vi "loop_with_message_channel.vi"() -> ()   [LabVIEW 2021]
uses:
  <extravilib>/ChannelInstances/Messenger-dbl/Write With Abort.vi
  <extravilib>/ChannelInstances/Messenger-dbl/Read With Abort.vi
  <extravilib>/ChannelInstances/Messenger-dbl/Instantiate.vi
  <extravilib>/ChannelInstances/Messenger-dbl/Endpoint.vi
  <extravilib>/ChannelInstances/Messenger-dbl.lvlib
panel:
  out "Waveform Chart 2":dbl(graph)
  out "Waveform Chart":dbl(graph)
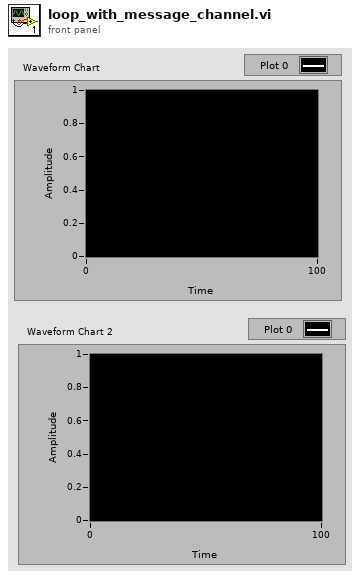
[diagram p1: front panel]
types:
  T1 = typedef "Messenger-dbl.lvlib/))Channel.ctl" = refnum<queue>
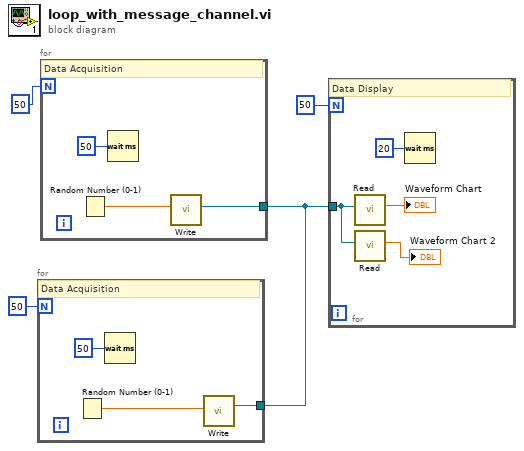
[diagram p0: block diagram]
diagram:
  n1 = for {
    N: 50 -> [_]
    tunnel: [w5] -> w1
    # "Data Acquisition"
    n2 = Random Number (0-1)() -> (number: 0 to 1=w6:dbl)
    n3 = Wait (ms)(milliseconds to wait=u32 50) -> ()  [unwired: 1 out]
    n4 = call <extravilib>:"Write.vi"("element"=w6) -> ("channel"=w5:T1)  [unwired: 8 in, 2 out]
  }
  n5 = for {
    N: 50 -> [_]
    tunnel: w1 -> [w8]
    # "Data Acquisition"
    n6 = Random Number (0-1)() -> (number: 0 to 1=w9:dbl)
    n7 = Wait (ms)(milliseconds to wait=u32 50) -> ()  [unwired: 1 out]
    n8 = call <extravilib>:"Write.vi"("element"=w9) -> ("channel"=w8:T1)  [unwired: 8 in, 2 out]
  }
  n9 = for {
    N: 50 -> [_]
    tunnel: w1 -> [w12]
    # "Data Display"
    n10 = call <extravilib>:"Read.vi"("channel"=w12) -> ("element"=→"Waveform Chart":dbl)  [unwired: 8 in, 2 out]
    n11 = call <extravilib>:"Read.vi"("channel"=w12) -> ("element"=→"Waveform Chart 2":dbl)  [unwired: 8 in, 2 out]
    n12 = Wait (ms)(milliseconds to wait=u32 20) -> ()  [unwired: 1 out]
  }
